vi "AgNA_Initialize and Config with Smoothing Aperture.vi"(8 "error in (no error)":errorcluster {"code" format="%.0x"}, 11 "NETAN":refnum<k15> caption="resource string") -> (0 "error out":errorcluster {"code" format="%.0x"}, 3 "instrument handle out":refnum<k15>)   [LabVIEW 2015]
uses:
  <instrlib>/Agilent NA/Agilent NA.lvlib
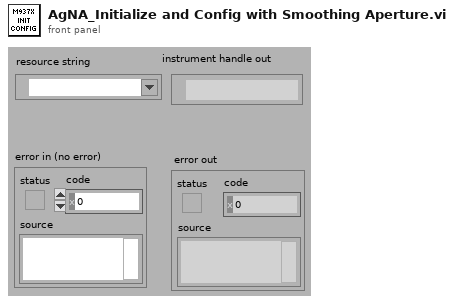
[diagram p1: front panel]
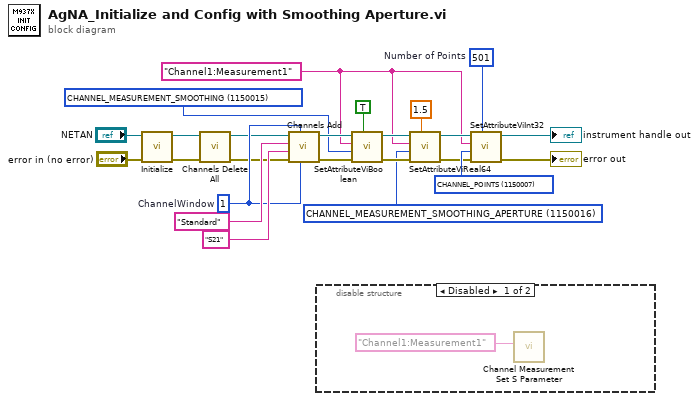
[diagram p0: block diagram]
diagram:
  w2 = u32 1150016 items=["CHANNEL_CW_FREQUENCY"=1150004, "CHANNEL_IF_BANDWIDTH"=1150005, "CHANNEL_MEASUREMENT_ELECTRICAL_DELAY_DISTANCE"=1150177, "CHANNEL_MEASUREMENT_ELECTRICAL_DELAY_TIME"=1150176, "CHANNEL_MEASUREMENT_ELECTRICAL_DELAY_VELOCITY_FACTOR"=1150180, "CHANNEL_MEASUREMENT_ELECTRICAL_DELAY_WAVE_GUIDE_CUT_OFF_FREQ"=1150179, "CHANNEL_MEASUREMENT_GROUP_DELAY_FREQUENCY"=1150172, "CHANNEL_MEASUREMENT_GROUP_DELAY_PERCENT"=1150174, "CHANNEL_MEASUREMENT_GROUP_DELAY_POINTS"=1150173, "CHANNEL_MEASUREMENT_MARKER_BANDWIDTH_THRESHOLD"=1150021, "CHANNEL_MEASUREMENT_MARKER_PEAK_EXCURSION"=1150024, "CHANNEL_MEASUREMENT_MARKER_STIMULUS"=1150025, "CHANNEL_MEASUREMENT_MARKER_TARGET_VALUE"=1150026, "CHANNEL_MEASUREMENT_SMOOTHING_APERTURE"=1150016, "CHANNEL_MEASUREMENT_TIME_DOMAIN_GATING_CENTER"=1150138, "CHANNEL_MEASUREMENT_TIME_DOMAIN_GATING_SPAN"=1150141, "CHANNEL_MEASUREMENT_TIME_DOMAIN_GATING_START"=1150142, "CHANNEL_MEASUREMENT_TIME_DOMAIN_GATING_STOP"=1150143, "CHANNEL_MEASUREMENT_TIME_DOMAIN_TRANSFORM_CENTER"=1150145, "CHANNEL_MEASUREMENT_TIME_DOMAIN_TRANSFORM_SPAN"=1150148, "CHANNEL_MEASUREMENT_TIME_DOMAIN_TRANSFORM_START"=1150149, "CHANNEL_MEASUREMENT_TIME_DOMAIN_TRANSFORM_STEP_RISE_TIME"=1150150, "CHANNEL_MEASUREMENT_TIME_DOMAIN_TRANSFORM_STOP"=1150151, "CHANNEL_MEASUREMENT_TIME_DOMAIN_WINDOW_IMPULSE_WIDTH"=1150152, "CHANNEL_MEASUREMENT_TIME_DOMAIN_WINDOW_KAISER_BETA"=1150153, "CHANNEL_MEASUREMENT_TRACE_REFERENCE_POSITION"=1150027, "CHANNEL_MEASUREMENT_TRACE_REFERENCE_VALUE"=1150028, "CHANNEL_MEASUREMENT_TRACE_Y_SCALE"=1150029, "CHANNEL_STIMULUS_RANGE_CENTER"=1150032, "CHANNEL_STIMULUS_RANGE_SPAN"=1150033, "CHANNEL_STIMULUS_RANGE_START"=1150034, "CHANNEL_STIMULUS_RANGE_STOP"=1150035, "CHANNEL_SWEEP_TIME"=1150010, "GUIDED_CALIBRATION__ADVANCED_IF_BAND_WIDTH"=1150171] ("AttributeID")
  w8 = u32 1150015 items=["CHANNEL_AVERAGING"=1150001, "CHANNEL_CORRECTION"=1150003, "CHANNEL_MEASUREMENT_LIMIT_ENABLE"=1150018, "CHANNEL_MEASUREMENT_MARKER_ENABLED"=1150022, "CHANNEL_MEASUREMENT_MARKER_MARKER_TRACK_ENABLED"=1150023, "CHANNEL_MEASUREMENT_SMOOTHING"=1150015, "CHANNEL_MEASUREMENT_TIME_DOMAIN_COUPLING_STATE"=1150136, "CHANNEL_MEASUREMENT_TIME_DOMAIN_GATING_ENABLE"=1150139, "CHANNEL_MEASUREMENT_TIME_DOMAIN_TRANSFORM_ENABLE"=1150146, "CHANNEL_MEASUREMENT_TRACE_ENABLE_TRACE_MAX"=1150182, "CHANNEL_PORT_EXTENSION_STATUS"=1150008, "CHANNEL_SOURCEPOWER_COUPLING"=1150031, "CHANNEL_SWEEP_TIME_AUTO"=1150011, "DISPLAY_ENABLED"=1150036, "GUIDED_CALIBRATION_ADVANCED_E_CAL_AUTO_ORIENTATION"=1150116, "SIMULATE"=1050005, "SYSTEM_POWER_ENABLED"=1150184, "SYSTEM_TRACE_ENABLED"=1150041, "WINDOW_STATE"=1150183, "WINDOW_TITLE_STATE"=1150132] ("AttributeID")
  w13 = 501  # Number of Points
  w19 = 1  # ChannelWindow
  w20 = u32 1150007 items=["CHANNEL_AVERAGING_FACTOR"=1150002, "CHANNEL_MEASUREMENT_ELECTRICAL_DELAY_MEDIUM"=1150178, "CHANNEL_MEASUREMENT_ELECTRICAL_DELAY_UNITS"=1150175, "CHANNEL_MEASUREMENT_FORMAT"=1150014, "CHANNEL_MEASUREMENT_LIMIT_NUMBER"=1150020, "CHANNEL_MEASUREMENT_TIME_DOMAIN_GATING_SHAPE"=1150140, "CHANNEL_MEASUREMENT_TIME_DOMAIN_GATING_TYPE"=1150144, "CHANNEL_MEASUREMENT_TIME_DOMAIN_PARAMETERS"=1150137, "CHANNEL_MEASUREMENT_TIME_DOMAIN_TRANSFORM_MODE"=1150147, "CHANNEL_MEASUREMENT_TRACE_MATH"=1150017, "CHANNEL_POINTS"=1150007, "CHANNEL_SWEEP_MODE"=1150009, "CHANNEL_SWEEP_TYPE"=1150012, "CHANNEL_TRIGGER_MODE"=1150013, "DISPLAY_ARRANGE_WINDOWS"=1150181, "SYSTEM_TIME_OUT_MILLISECONDS"=1150040, "TRIGGER_SOURCE"=1150042, "WINDOW_SIZE"=1150133, "WINDOW_TABLE"=1150134] ("AttributeID")
  w3 = "Channel1:Measurement1" ("RepCapIdentifier")
  n1 = call <instrlib>:"Initialize.vi"("error in (no error)"="error in (no error)", "resource name"="NETAN") -> ("error out"=w16:errorcluster, "instrument handle out"=w17:refnum<k15>)  [unwired: 8 in]
  n2 = call <instrlib>:"Channels Delete All.vi"("error in (no error)"=w16, "instrument handle"=w17) -> ("error out"=w15:errorcluster, "instrument handle out"=w14:refnum<k15>)  [unwired: 8 in]
  n3 = call <instrlib>:"Channels Add.vi"("WindowNumber"=w19, "ChannelNumber"=w19, "error in (no error)"=w15, "ChannelParameter"="S21", "ChannelType"="Standard", "instrument handle"=w14) -> ("error out"=w9:errorcluster, "instrument handle out"=w18:refnum<k15>)  [unwired: 3 in, 1 out]
  n4 = disable-structure shown="Disabled" {
    frame Disabled {
      n5 = call <instrlib>:"Channel Measurement Set S Parameter.vi"("RepCapIdentifier"="Channel1:Measurement1") -> ()  [unwired: 9 in, 2 out]
    }
    frame Enabled {
    }
  }
  n6 = call <instrlib>:"SetAttributeViBoolean.vi"("AttributeValue (Off)"=TRUE, "error in (no error)"=w9, "AttributeID"=w8, "RepCapIdentifier"=w3, "instrument handle"=w18) -> ("error out"=w5:errorcluster, "instrument handle out"=w10:refnum<k15>)  [unwired: 5 in]
  n7 = call <instrlib>:"SetAttributeViReal64.vi"("AttributeValue"=1.5, "error in (no error)"=w5, "AttributeID"=w2, "RepCapIdentifier"=w3, "instrument handle"=w10) -> ("error out"=w4:errorcluster, "instrument handle out"=w6:refnum<k15>)  [unwired: 5 in]
  n8 = call <instrlib>:"SetAttributeViInt32.vi"("AttributeValue"=w13, "error in (no error)"=w4, "AttributeID"=w20, "RepCapIdentifier"=w3, "instrument handle"=w6) -> ("error out"=→"error out":errorcluster, "instrument handle out"=→"instrument handle out":refnum<k15>)  [unwired: 5 in]
